vi "AutoSetUpMetodo.vi"(8 "error in (no error)":errorcluster, 10 "VISA resource name":refnum<visa-resource-name>, 11 "Osciloscope in":refnum<class "Osciloscope.lvclass">) -> (0 "error out":errorcluster, 2 "VISA resource name out":refnum<visa-resource-name>, 3 "Osciloscope out":refnum<class "Osciloscope.lvclass">)   [LabVIEW 2020, in "Osciloscope.lvclass"]
uses:
  Osciloscope.lvclass
  Osciloscope.lvclass/Osciloscope.ctl
  <instrlib>/Tektronix TDS 200 1000 2000 Series/Tektronix TDS 200 1000 2000 Series.lvlib
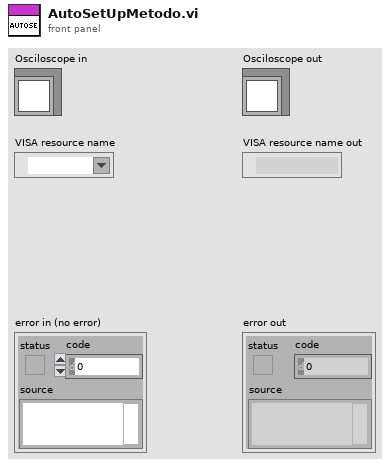
[diagram p1: front panel]
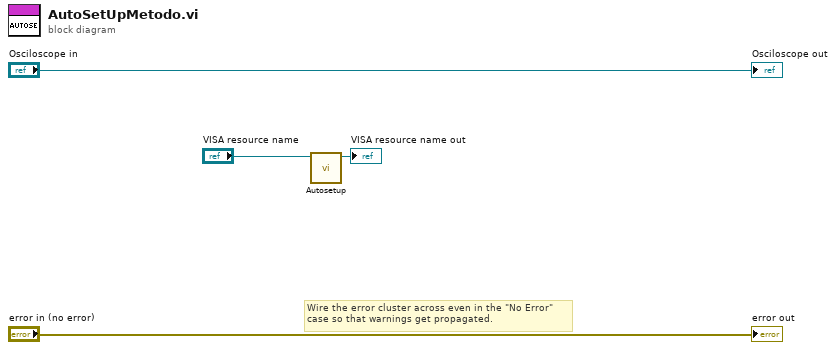
[diagram p0: block diagram]
diagram:
  # "Wire the error cluster across even in the \"No Error\"\ncase so that warnings get propagated."
  n1 = call <instrlib>:"Autosetup.vi"("VISA resource name"="VISA resource name") -> ("VISA resource name out"=→"VISA resource name out":refnum<visa-resource-name>)  [unwired: 9 in, 1 out]
  "error out" <- "error in (no error)"
  "Osciloscope out" <- "Osciloscope in"
